vi "SEND RECEIVER ISP310 PROGRAM.vi"(0 "VISA resource name in":refnum<visa-resource-name>, 5 "PROGRAM":string(combo)="1", 9 "CHECKSUM IN":string, 11 "error in (no error)":errorcluster) -> (4 "VISA resource name out":refnum<visa-resource-name>, 6 "FILE PROGRAM":string, 8 "CHECK SUM OUT":string, 10 "CHECKSUM ?":bool, 15 "error out":errorcluster)   [LabVIEW 2017]
uses:
  <vilib>/Instr/_visa.llb/VISA Flush IO Buffer Mask.ctl
  <vilib>/Instr/_visa.llb/VISA Configure Serial Port (Instr).vi
panel:
  # "#W03\n#END\n#NAM:180208-2_BA8_STs\n#SUM:002E43EE"
  # "CMD: #W01/A"
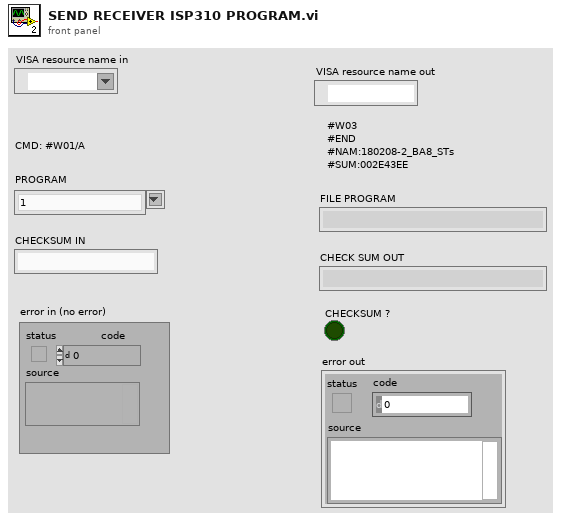
[diagram p1: front panel]
types:
  T1 = typedef "VISA Flush IO Buffer Mask.ctl" = u16
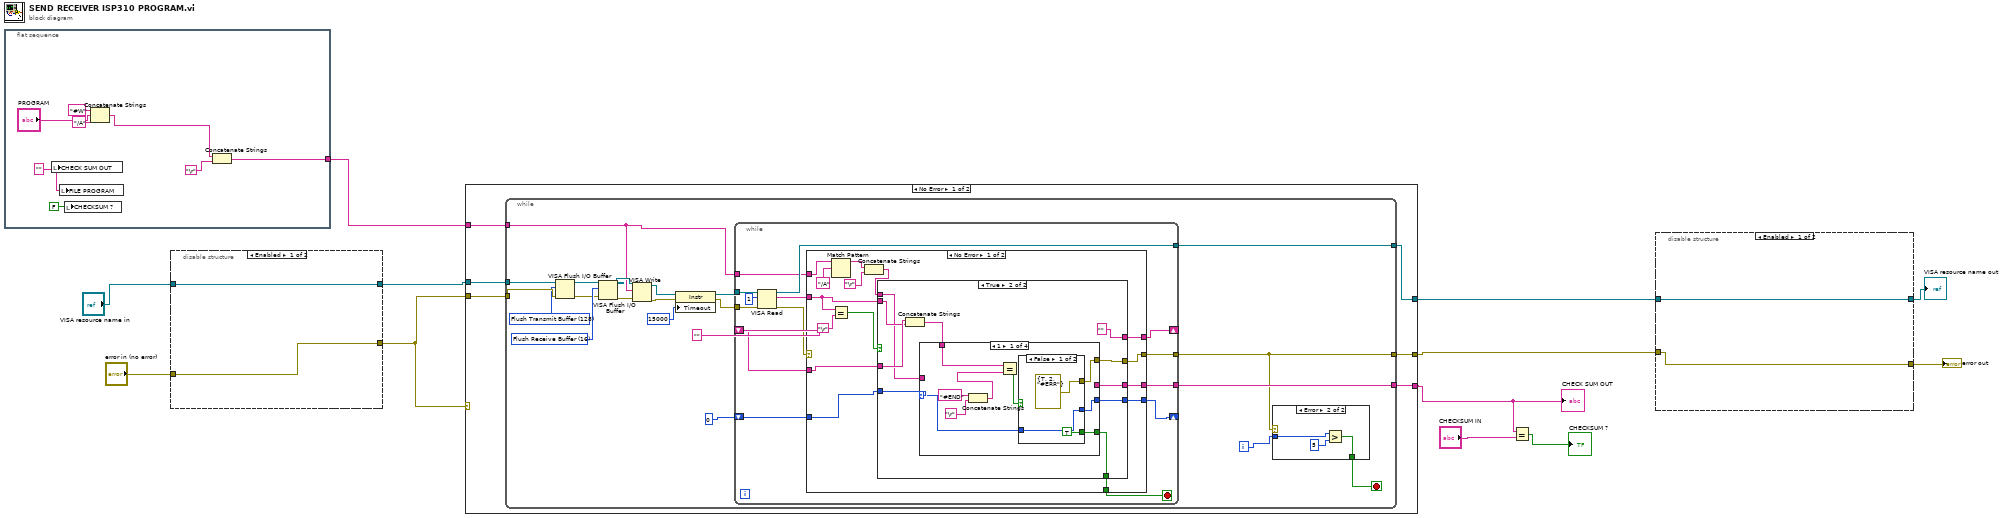
[diagram p0: block diagram]
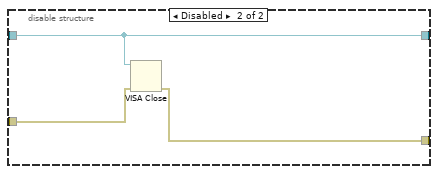
[diagram p2: hidden frame]
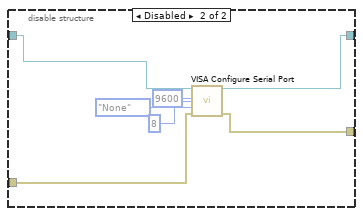
[diagram p3: hidden frame]
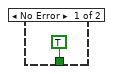
[diagram p4: hidden frame]
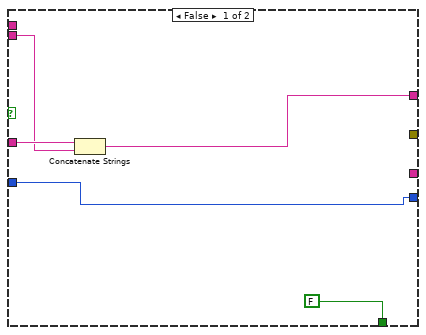
[diagram p5: hidden frame]
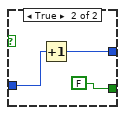
[diagram p6: hidden frame]
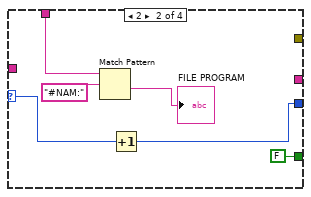
[diagram p7: hidden frame]
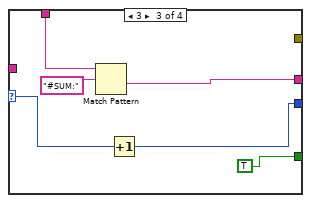
[diagram p8: hidden frame]
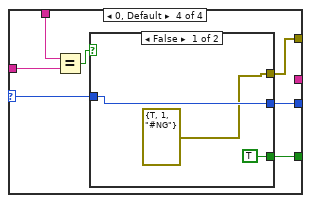
[diagram p9: hidden frame]
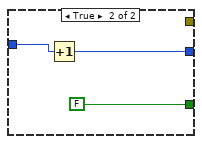
[diagram p10: hidden frame]
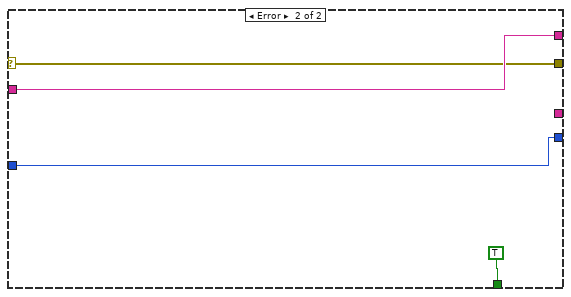
[diagram p11: hidden frame]
diagram:
  n1 = flat-sequence {
    tunnel: [w19] -> w9
    frame #0 {
      w18 = ""
      n2 = local write "CHECK SUM OUT"(w18) -> ()
      n3 = local write "FILE PROGRAM"(w18) -> ()
      n4 = local write "CHECKSUM ?"(FALSE ("CHECKSUM ?")) -> ()
      n5 = Concatenate Strings("#W" ("string"), "PROGRAM", "/A" ("string")) -> (w14:string)
      n6 = Concatenate Strings(w14, "\r") -> (w19:string)
    }
  }
  n7 = disable-structure shown="Enabled" {
    disable-tunnel: [w22 w28] -> w12
    disable-tunnel: [w21 w29] -> w5
    disable-tunnel: "error in (no error)" -> [w22 w24]
    disable-tunnel: "VISA resource name in" -> [w21 w23]
    frame Enabled {
    }
    frame Disabled {
      n8 = call-poly "VISA Configure Serial Port"("VISA resource name"=w23, "baud rate (9600)"=u32 9600, "data bits (8)"=u16 8, "parity (0:none)"=enum16{"None", "Odd", "Even", "Mark", "Space"}."None", "error in (no error)"=w24) -> ("VISA resource name out"=w29:refnum<visa-resource-name>, "error out"=w28:errorcluster)  [unwired: 9 in]
    }
  }
  n9 = case shown="No Error" w12 {
    tunnel: w12 -> [w34 w150]
    tunnel: w5 -> [w35 w149]
    tunnel: [w33 w150] -> w11
    tunnel: [w32 w149] -> w10
    tunnel: w9 -> [w31 _]
    tunnel: [w30 _] -> w4
    frame No Error {
      n10 = while {
        tunnel: w34 -> [w54]
        tunnel: w35 -> [w55]
        tunnel: [w38] -> w33
        tunnel: [w44] -> w32
        tunnel: w31 -> [w41]
        tunnel: [w39] -> w30
        i -> [w36]
        stop <- w37 stop-if-true
        w53 = T1 128 items=["Flush Receive Buffer"=16, "Write Transmit Buffer to Device"=32, "Flush Receive Buffer (No I/O)"=64, "Flush Transmit Buffer"=128] ("Mask")
        w56 = T1 16 items=["Flush Receive Buffer"=16, "Write Transmit Buffer to Device"=32, "Flush Receive Buffer (No I/O)"=64, "Flush Transmit Buffer"=128] ("Mask")
        n11 = VISA Flush I/O Buffer(VISA resource name=w55, mask (16)=w53, error in (no error)=w54) -> (VISA resource name out=w50:refnum<visa-resource-name>, error out=w49:errorcluster)
        n12 = VISA Flush I/O Buffer(VISA resource name=w50, mask (16)=w56, error in (no error)=w49) -> (VISA resource name out=w52:refnum<visa-resource-name>, error out=w51:errorcluster)
        n13 = VISA Write(VISA resource name=w52, write buffer=w41, error in (no error)=w51) -> (VISA resource name out=w47:refnum<visa-resource-name>, error out=w42:errorcluster)  [unwired: 1 out]
        n14 = property class="Instr"(reference=w47, error in=w42, "Timeout"=u32 15000 ("General Settings:Timeout Value")) -> (reference out=w48:refnum<visa-resource-name>, error out=w43:errorcluster)
        n15 = while {
          tunnel: w48 -> [w74]
          tunnel: w43 -> [w73]
          shift-right: [w67] -> _
          shift-left: "" -> [w68]
          tunnel: [w66] -> w38
          tunnel: [w65] -> w44
          tunnel: w41 -> [w64]
          shift-right: [w62] -> _
          shift-left: 0 -> [w63]
          tunnel: [w61] -> w39
          stop <- w69 stop-if-true
          n16 = VISA Read(VISA resource name=w74, byte count=u32 1, error in (no error)=w73) -> (VISA resource name out=w65:refnum<visa-resource-name>, read buffer=w70:string, error out=w71:errorcluster)  [unwired: 1 out]
          n17 = case shown="No Error" w71 {
            selector: w71 -> [_ w146]
            tunnel: w70 -> [w80 _]
            tunnel: [w85 TRUE] -> w69
            tunnel: w68 -> [w81 w147]
            tunnel: [w88 w147] -> w67
            tunnel: [w83 w146] -> w66
            tunnel: w64 -> [w79 _]
            tunnel: w63 -> [w86 w145]
            tunnel: [w84 w145] -> w62
            tunnel: [w82 _] -> w61
            frame No Error {
              n18 = Match Pattern(string=w79, regular expression="/A") -> (before substring=w77:string)  [unwired: 1 in, 3 out]
              n19 = Equal?(x=w80, y="\r") -> (x = y?=w89:bool)
              n20 = Concatenate Strings(w77, "\r") -> (w75:string)
              n21 = case shown="True" w89 {
                tunnel: w81 -> [w94 w104]
                tunnel: w80 -> [w93 w103]
                tunnel: [w92 ""] -> w88
                tunnel: w75 -> [_ w101]
                tunnel: w86 -> [w90 w100]
                tunnel: [FALSE w99] -> w85
                tunnel: [w90 w98] -> w84
                tunnel: [_ w97] -> w83
                tunnel: [_ w96] -> w82
                frame False {
                  n22 = Concatenate Strings(w94, w93) -> (w92:string)
                }
                frame True {
                  n23 = Concatenate Strings(w104, w103) -> (w102:string)
                  n24 = case shown="1" w100 {
                    selector: w100 -> [w106 w125 w131 w134]
                    tunnel: w102 -> [w113 w122 w128 w138]
                    tunnel: w101 -> [_ _ _ w137]
                    tunnel: [w108 FALSE TRUE w135] -> w99
                    tunnel: [w107 w124 w130 w133] -> w98
                    tunnel: [w105 _ _ w132] -> w97
                    tunnel: [_ _ w126 _] -> w96
                    frame 1 {
                      n25 = Concatenate Strings("#END", "\r") -> (w110:string)
                      n26 = Equal?(x=w113, y=w110) -> (x = y?=w109:bool)
                      n27 = case shown="False" w109 {
                        tunnel: [TRUE FALSE] -> w108
                        tunnel: [w116 w118] -> w107
                        tunnel: w106 -> [w116 w117]
                        tunnel: [errorcluster {"status"=TRUE, "code"=2, "source"="#ERR"} ("error constant") _] -> w105
                        frame False {
                        }
                        frame True {
                          n28 = Increment(x=w117) -> (x+1=w118:i32)
                        }
                      }
                    }
                    frame 2 {
                      n29 = Match Pattern(string=w122, regular expression="#NAM:") -> (after substring=→"FILE PROGRAM":string)  [unwired: 1 in, 3 out]
                      n30 = Increment(x=w125) -> (x+1=w124:i32)
                    }
                    frame 3 {
                      n31 = Match Pattern(string=w128, regular expression="#SUM:") -> (after substring=w126:string)  [unwired: 1 in, 3 out]
                      n32 = Increment(x=w131) -> (x+1=w130:i32)
                    }
                    frame 0, Default {
                      n33 = Equal?(x=w138, y=w137) -> (x = y?=w136:bool)
                      n34 = case shown="False" w136 {
                        tunnel: [TRUE FALSE] -> w135
                        tunnel: w134 -> [w141 w143]
                        tunnel: [w141 w142] -> w133
                        tunnel: [errorcluster {"status"=TRUE, "code"=1, "source"="#NG"} ("error constant") _] -> w132
                        frame False {
                        }
                        frame True {
                          n35 = Increment(x=w143) -> (x+1=w142:i32)
                        }
                      }
                    }
                  }
                }
              }
            }
            frame Error {
            }
          }
        }
        n36 = case shown="Error" w38 {
          tunnel: [TRUE w59] -> w37
          tunnel: w36 -> [_ w58]
          frame No Error {
          }
          frame Error {
            n37 = Greater?(x=w58, y=5) -> (0:w59:bool)
          }
        }
      }
    }
    frame Error {
    }
  }
  "CHECK SUM OUT" <- w4
  n38 = Equal?(x=w4, y="CHECKSUM IN") -> (x = y?=→"CHECKSUM ?":bool)
  n39 = disable-structure shown="Enabled" {
    disable-tunnel: w11 -> [w152 w155]
    disable-tunnel: w10 -> [w151 w153]
    disable-tunnel: [w152 w154] -> w8
    disable-tunnel: [w151 w153] -> w1
    frame Enabled {
    }
    frame Disabled {
      n40 = VISA Close(VISA resource name=w153, error in (no error)=w155) -> (error out=w154:errorcluster)
    }
  }
  "error out" <- w8
  "VISA resource name out" <- w1
